vi "Error Code to Message.vi"(10 "Error Code (0)":i32) -> (2 "Error Message":string)   [LabVIEW 2020, in "ADCMT 6240.lvlib"]
doc: "This VI converts an error code into message character string."
uses:
  ADCMT 6240.lvlib
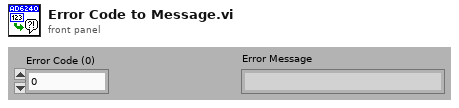
[diagram p1: front panel]
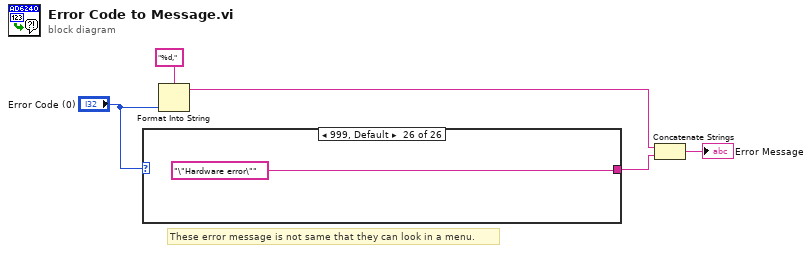
[diagram p0: block diagram]
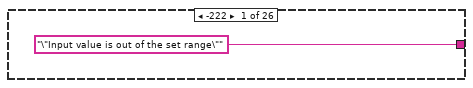
[diagram p2: hidden frame]
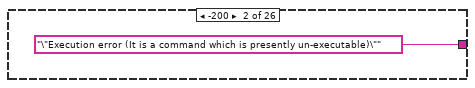
[diagram p3: hidden frame]
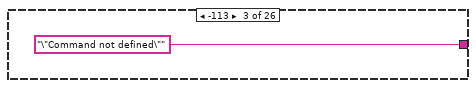
[diagram p4: hidden frame]
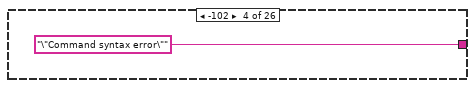
[diagram p5: hidden frame]
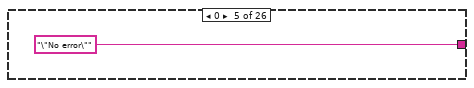
[diagram p6: hidden frame]
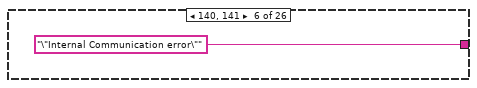
[diagram p7: hidden frame]
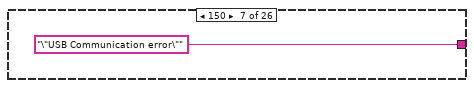
[diagram p8: hidden frame]
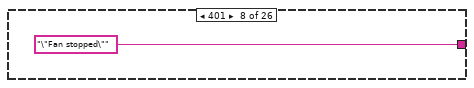
[diagram p9: hidden frame]
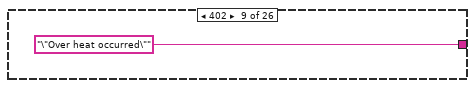
[diagram p10: hidden frame]
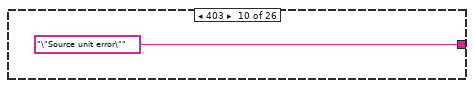
[diagram p11: hidden frame]
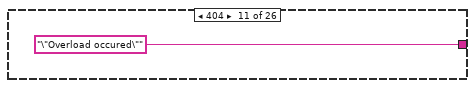
[diagram p12: hidden frame]
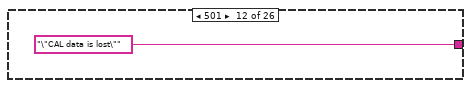
[diagram p13: hidden frame]
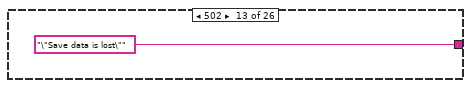
[diagram p14: hidden frame]
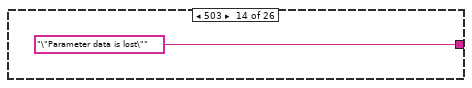
[diagram p15: hidden frame]
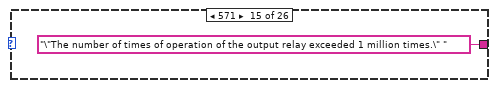
[diagram p16: hidden frame]
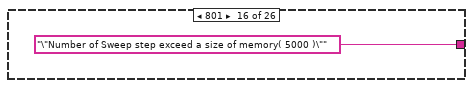
[diagram p17: hidden frame]
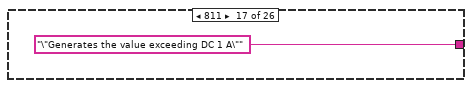
[diagram p18: hidden frame]
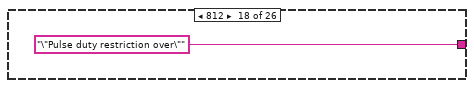
[diagram p19: hidden frame]
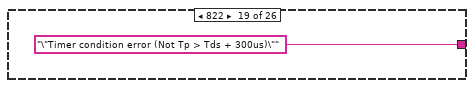
[diagram p20: hidden frame]
diagram:
  # "These error message is not same that they can look in a menu."
  n1 = case shown="999, Default" "Error Code (0)" {
    tunnel: ["\"Input value is out of the set range\"" "\"Execution error (It is a command which is presently un-executable)\"" "\"Command not defined\"" "\"Command syntax error\"" "\"No error\"" "\"Internal Communication error\"" "\"USB Communication error\"" "\"Fan stopped\"" "\"Over heat occurred\"" "\"Source unit error\"" "\"Overload occured\"" "\"CAL data is lost\"" "\"Save data is lost\"" "\"Parameter data is lost\"" "\"The number of times of operation of the output relay exceeded 1 million times.\" " "\"Number of Sweep step exceed a size of memory( 5000 )\"" "\"Generates the value exceeding DC 1 A\"" "\"Pulse duty restriction over\"" "\"Timer condition error (Not Tp > Tds + 300us)\"" "\"Timer condition error (Not Tp > Td + 300us)\"" "\"Timer condition error (Not Tp > Tds + Tw + 300us)\"" "\"Timer condition error (Not Tp > Tds)\"" "\"Timer condition error (Not Tp <= 600ms)\"" "\"Disabled status by Interlock\"" "\"Calibration data error\"" "\"Hardware error\""] -> w3
    frame -222 {
    }
    frame -200 {
    }
    frame -113 {
    }
    frame -102 {
    }
    frame 0 {
    }
    frame 140, 141 {
    }
    frame 150 {
    }
    frame 401 {
    }
    frame 402 {
    }
    frame 403 {
    }
    frame 404 {
    }
    frame 501 {
    }
    frame 502 {
    }
    frame 503 {
    }
    frame 571 {
    }
    frame 801 {
    }
    frame 811 {
    }
    frame 812 {
    }
    frame 822 {
    }
    frame 823 {
    }
    frame 824 {
    }
    frame 825 {
    }
    frame 828 {
    }
    frame 831 {
    }
    frame 855 {
    }
    frame 999, Default {
    }
  }
  n2 = Format Into String(format string="%d,", "Error Code (0)") -> (resulting string=w2:string)  [unwired: 2 in, 1 out]
  n3 = Concatenate Strings(w2, w3) -> (→"Error Message":string)
